vi "Determine If Left or Right Sector.vi"(11 "X Pixel Location":u16) -> (3 "Right Sector?":bool)   [LabVIEW 2013]
uses:
  Globals/Pixel Location Global.vi
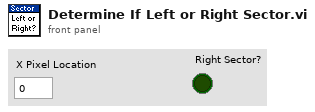
[diagram p1: front panel]
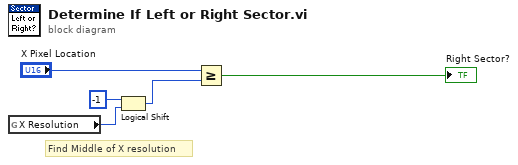
[diagram p0: block diagram]
diagram:
  # "Find Middle of X resolution"
  n1 = global read "Pixel Location Global.vi" "X Resolution"() -> (w3:u16)
  n2 = Logical Shift(y=i16 -1, x=w3) -> (x << y=w1:u16)
  n3 = Greater Or Equal?(x="X Pixel Location", y=w1) -> (x >= y?=→"Right Sector?":bool)
